vi "Launcher.vi"() -> ()   [LabVIEW 2019]
doc: "This VI launces the Command design pattern and tells the agent (Invoker) to send Buy Stock Order and Sell Stock Order (Concrete Commands) to StockTrade (Reciever). StockTrade controls the Display String Indicator so that the interactions are visible. The Order class (Command) provides the interface for Buy Stock Order and Sell Stock Order to override."
uses:
  Agent/Agent.lvclass
  Stock Trader/Stock Trader.lvclass
  Orders/Buy Stock Order/Buy Stock Order.lvclass
  C:/Users/Tiba/Desktop/Command Pattern 2014/Command Pattern 2014/Order/Order.lvclass
  Orders/Sell Stock Order/Sell Stock Order.lvclass
panel:
  out "Display String":string
  in  "Clear":bool
  in  "Sell":bool
  in  "Buy":bool
  out "error out":errorcluster
  in  "stop":bool
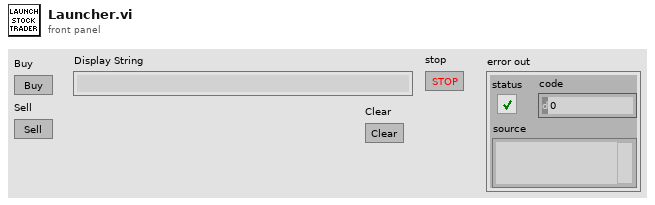
[diagram p1: front panel]
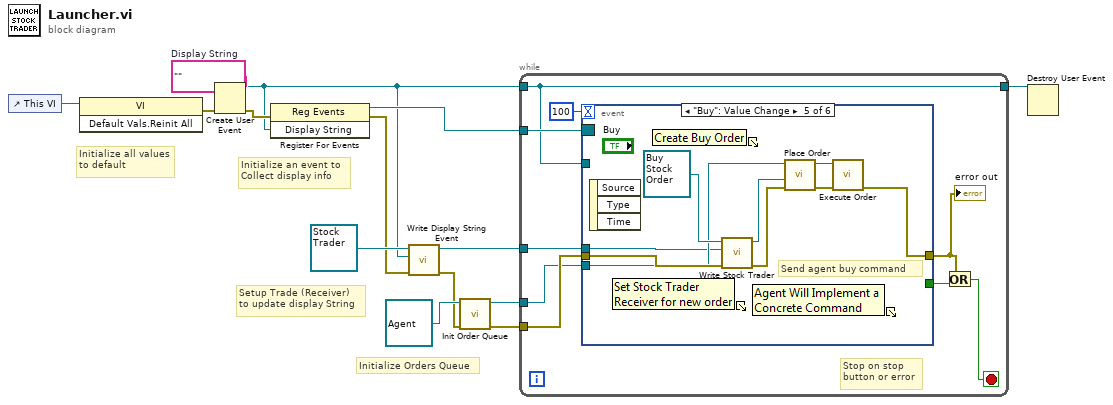
[diagram p0: block diagram]
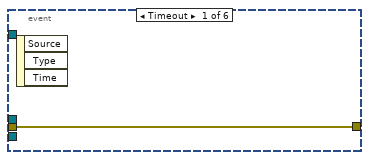
[diagram p2: hidden frame]
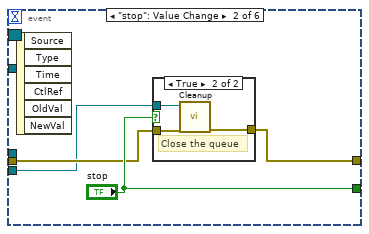
[diagram p3: hidden frame]
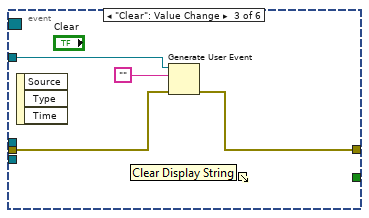
[diagram p5: hidden frame]
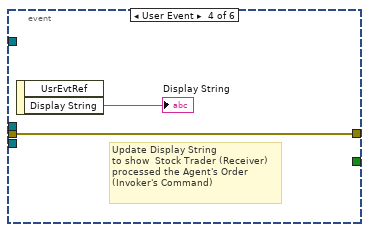
[diagram p6: hidden frame]
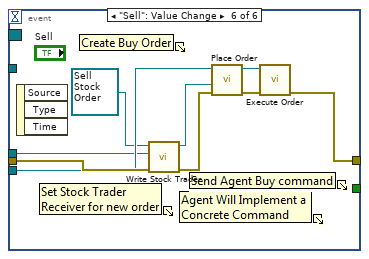
[diagram p7: hidden frame]
diagram:
  w13 = ""  # Display String
  # "Initialize Orders Queue"
  # "Setup Trade (Receiver)\nto update display String"
  # "Initialize all values\nto default"
  # "Initialize an event to \nCollect display info"
  n1 = control-ref of="This VI"() -> (w14:refnum<vi>)
  n2 = invoke class="VI" method="Default Vals.Reinit All"(reference=w14) -> (error out=w12:errorcluster)  [unwired: 2 in, 2 out]
  n3 = Create User Event(user event datatype=w13, error in=w12) -> (user event=w1:refnum<user-event>, error out=w10:errorcluster)
  n4 = register-events(error in=w10, w1) -> (reference out=w9:refnum<event-registration>, error out=w2:errorcluster)  [unwired: 1 in]
  n5 = call-dynamic "Write Display String Event.vi"("error in (no error)"=w2, "Display String Event"=w1, "Stock Trader in"=refnum<class "Stock Trader.lvclass"> refnum ("Stock Trader.lvclass")) -> ("error out"=w3:errorcluster, "Stock Trader out"=w4:refnum<class "Stock Trader.lvclass">)  [unwired: 7 in]
  n6 = call-dynamic "Init Order Queue.vi"("error in (no error)"=w3, "Agent in"=refnum<class "Agent.lvclass"> refnum ("Agent.lvclass")) -> ("error out"=w6:errorcluster, "Agent out"=w7:refnum<class "Agent.lvclass">)  [unwired: 7 in, 1 out]
  n7 = while {
    tunnel: w1 -> [w15]
    tunnel: [w15] -> w11
    tunnel: w9 -> [w23]
    tunnel: w7 -> [w20]
    tunnel: w6 -> [w21]
    tunnel: w4 -> [w19]
    stop <- w16 stop-if-true
    # "Stop on stop \nbutton or error"
    n8 = event shown="[4] \"Buy\": Value Change" {
      selector: w23 -> [_ _ _ _ _ _]
      dyn-events: _ -> [_ _ _ _ _ _]
      timeout: 100 -> [_ _ _ _ _ _]
      tunnel: w21 -> [w24 w27 w36 w37 w47 w56]
      tunnel: w20 -> [_ w25 _ _ w42 w52]
      tunnel: w19 -> [_ _ _ _ w39 w50]
      tunnel: [_ "stop" _ _ _ _] -> w18
      tunnel: [w24 w26 w35 w37 w46 w55] -> w17
      tunnel: w15 -> [_ _ w33 _ _ _]
      event Timeout {
        n9 = event-data() -> ()  [unwired: 1 in, 3 out]
      }
      event "stop": Value Change {
        n10 = event-data() -> ()  [unwired: 1 in, 6 out]
        n11 = case shown="True" "stop" {
          tunnel: w27 -> [w29 w32]
          tunnel: [w29 w31] -> w26
          tunnel: w25 -> [_ w30]
          frame False {
          }
          frame True {
            # "Close the queue"
            n12 = call "Cleanup.vi"("error in (no error)"=w32, "Agent_Inv In"=w30) -> ("error out"=w31:errorcluster)  [unwired: 9 in]
          }
        }
      }
      event "Clear": Value Change {
        n13 = event-data() -> ()  [unwired: 1 in, 3 out]
        n14 = Generate User Event(user event=w33, event data cluster="", error in=w36) -> (error out=w35:errorcluster)  [unwired: 1 in, 1 out]
      }
      event User Event {
        # "Update Display String\nto show  Stock Trader (Receiver)\nprocessed the Agent's Order\n(Invoker's Command)"
        n15 = event-data() -> ("Display String"=→"Display String":string)  [unwired: 1 in, 1 out]
      }
      event "Buy": Value Change {
        # "Send agent buy command"
        n16 = event-data() -> ()  [unwired: 1 in, 3 out]
        n17 = call-dynamic "Write Stock Trader.vi"("error in (no error)"=w47, "Stock Trader"=w39, "Order in"=refnum<class "Buy Stock Order.lvclass"> refnum ("Buy Stock Order.lvclass")) -> ("error out"=w44:errorcluster, "Order out"=w40:refnum<class "Buy Stock Order.lvclass">)  [unwired: 7 in]
        n18 = call "Place Order.vi"("error in (no error)"=w44, "Order To Place"=w40, "Agent In"=w42) -> ("error out"=w45:errorcluster, "Agent Out"=w41:refnum<class "Agent.lvclass">)  [unwired: 7 in]
        n19 = call-dynamic "Execute Order.vi"("error in (no error)"=w45, "Agent in"=w41) -> ("error out"=w46:errorcluster)  [unwired: 6 in, 3 out]
      }
      event "Sell": Value Change {
        n20 = event-data() -> ()  [unwired: 1 in, 3 out]
        n21 = call-dynamic "Write Stock Trader.vi"("error in (no error)"=w56, "Stock Trader"=w50, "Order in"=refnum<class "Sell Stock Order.lvclass"> refnum ("Sell Stock Order.lvclass")) -> ("error out"=w53:errorcluster, "Order out"=w49:refnum<class "Sell Stock Order.lvclass">)  [unwired: 7 in]
        n22 = call "Place Order.vi"("error in (no error)"=w53, "Order To Place"=w49, "Agent In"=w52) -> ("error out"=w54:errorcluster, "Agent Out"=w48:refnum<class "Agent.lvclass">)  [unwired: 7 in]
        n23 = call-dynamic "Execute Order.vi"("error in (no error)"=w54, "Agent in"=w48) -> ("error out"=w55:errorcluster)  [unwired: 6 in, 3 out]
      }
    }
    "error out" <- w17
    n24 = Or(x=w17, y=w18) -> (x .or. y?=w16:bool)
  }
  n25 = Destroy User Event(user event=w11) -> ()  [unwired: 1 in, 1 out]
